vi "Acquire and Save.vi"(8 "error in (no error)":errorcluster, 11 "ATS9462 Class in":refnum<class "ATS9462 Class.lvclass">) -> (0 "error out":errorcluster, 3 "ATS9462 Class out":refnum<class "ATS9462 Class.lvclass">)   [LabVIEW 2014, in "ATS9462 Class.lvclass"]
uses:
  ATS9462 Class.lvclass
  DAQ Class.lvclass
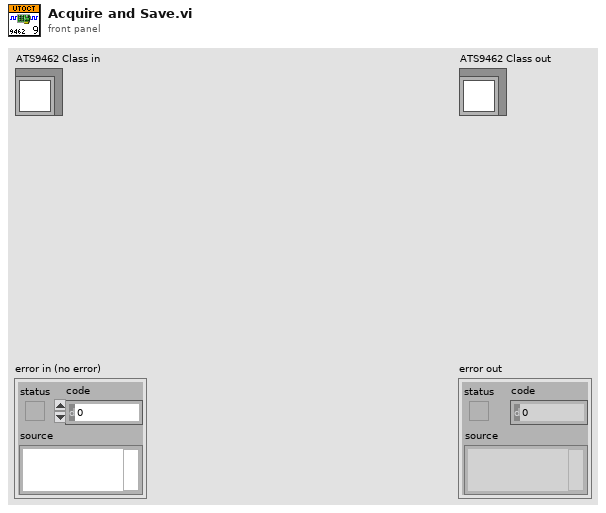
[diagram p1: front panel]
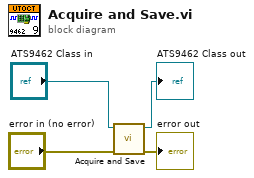
[diagram p0: block diagram]
diagram:
  n1 = call-parent "Acquire and Save.vi"("error in (no error)"="error in (no error)", "DAQ Class in"="ATS9462 Class in") -> ("error out"=→"error out":errorcluster, "DAQ Class out"=→"ATS9462 Class out":refnum<class "ATS9462 Class.lvclass">)  [unwired: 8 in]
